vi "probe_calibration.vi"(6 "z offset":sgl=2500.0, 8 "Calibration task":T1, 10 "World light positions":T2 format="%#.1f", 11 "Output pose":dbl[][](array[numeric])) -> (2 "Probe calibration":T2 format="%#.1f")   [LabVIEW 2013]
uses:
  probe_calibration.ctl
  calibration_task.ctl
  <vilib>/Analysis/baseanly.llb/A x Vector.vi
  utilities/labview/norm_vec_single.vi
  <vilib>/Analysis/baseanly.llb/Real A x B.vi
  utilities/labview/norm_vec.vi
  <vilib>/Analysis/baseanly.llb/Real Inverse Matrix.vi
  <vilib>/Analysis/NI_AALBase.lvlib
panel:
  out "Basis":dbl[][](array[numeric])
  # "Construct light calibration from the current light positions.  For the tip lights, this is an initial approximation of the light positions with an arbitrary coordinates based purely on the light locations.  This calibrates for the relative locations of the lights (minimizing triad error.)  With handle lights, the tip coordinates are used to construct the handle coordinates at a fixed Z offset, insuring alignment of the two coordinate systems and eliminating the need for the pivot calibration procedures.  The manipulator must be homed by bottoming it out to force the handle pose into a known relation to the output pose."
  # "This is the offset in microns from light 0  to the origin."
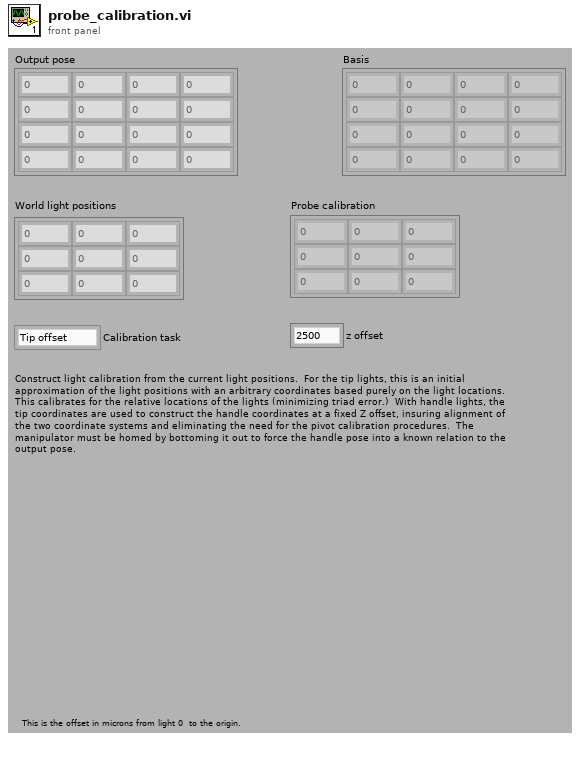
[diagram p1: front panel]
types:
  T1 = typedef "calibration_task.ctl" = enum16{"Tip offset", "RCM offset", "Tip lights", "Handle lights"}
  T2 = typedef "probe_calibration.ctl" = sgl[][]
  T3 = typedef "NI_Matrix.lvlib/RealMatrix.ctl" = dbl[][]
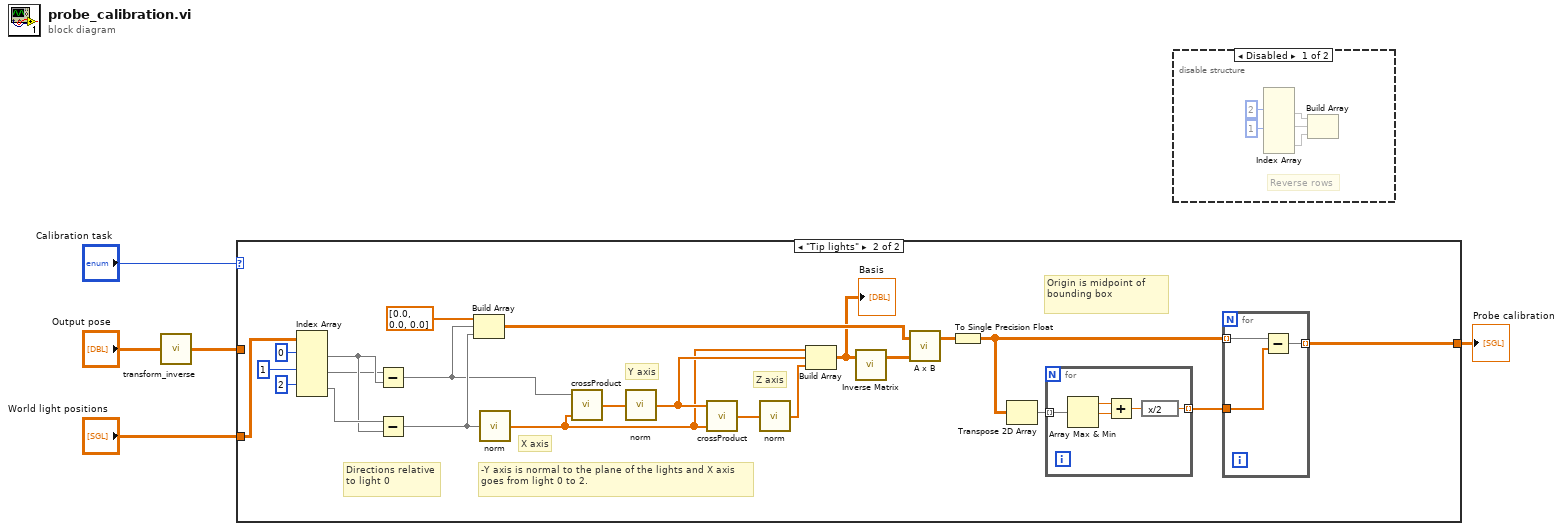
[diagram p0: block diagram]
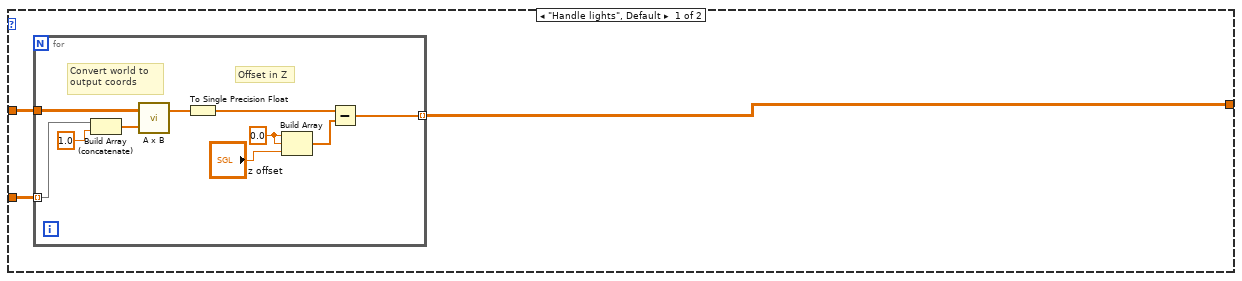
[diagram p3: hidden frame]
diagram:
  n1 = call "transform_inverse.vi"("Transform"="Output pose") -> ("Inverse transform"=w1:T3)
  n2 = case shown="\"Tip lights\"" "Calibration task" {
    tunnel: [w6 w21] -> w5
    tunnel: "World light positions" -> [w8 w27]
    tunnel: w1 -> [w7 _]
    frame "Handle lights", Default {
      n3 = for {
        tunnel: w8 -> [w14] mode=indexing
        tunnel: [w18] -> w6 mode=indexing
        tunnel: w7 -> [w11]
        w16 = sgl 0.0 ("element")
        # "Offset in Z"
        # "Convert world to \noutput coords"
        n4 = Build Array (concatenate)(w14, sgl 1.0) -> (w12:sgl[])
        n5 = call-poly <vilib>:"A x B.vi"("Vector"=w12, "A"=w11) -> ("A x Vector"=w10:dbl[])  [unwired: 1 out]
        n6 = To Single Precision Float(number=w10) -> (single precision float=w9:sgl[])
        n7 = Build Array(w16, w16, "z offset") -> (w15:sgl[])
        n8 = Subtract(x=w9, y=w15) -> (x-y=w18:sgl[])
      }
    }
    frame "Tip lights" {
      # "Origin is midpoint of bounding box"
      # "-Y axis is normal to the plane of the lights and X axis goes from light 0 to 2."
      # "Directions relative to light 0"
      # "Z axis"
      # "Y axis"
      # "X axis"
      n9 = Index Array(array=w27, index (row) #1=0 ("index (row)"), index (row) #2=1 ("index (row)"), index (row) #3=2 ("index (row)")) -> (element #1=w37:sgl[], element #2=w36:sgl[], element #3=w38:sgl[])  [unwired: 3 in]
      n10 = Subtract(x=w36, y=w37) -> (x-y=w20:sgl[])
      n11 = Subtract(x=w38, y=w37) -> (x-y=w31:sgl[])
      n12 = Build Array(dbl[] [0.0, 0.0, 0.0] ("normalized vector"), w20, w31) -> (w30:dbl[][])
      n13 = call-poly "norm.vi"("vector"=w31) -> ("normalized vector"=w19:sgl[])  [unwired: 4 out]
      n14 = call "crossProduct.vi"("B"=w19, "A"=w20) -> ("A x B"=w35:dbl[])  [unwired: 3 out]
      n15 = call-poly "norm.vi"("vector"=w35) -> ("normalized vector"=w23:dbl[])  [unwired: 4 out]
      n16 = call "crossProduct.vi"("B"=w19, "A"=w23) -> ("A x B"=w34:dbl[])  [unwired: 3 out]
      n17 = call-poly "norm.vi"("vector"=w34) -> ("normalized vector"=w33:dbl[])  [unwired: 4 out]
      n18 = Build Array(w19, w23, w33) -> (w22:dbl[][])
      "Basis" <- w22
      n19 = call-poly <vilib>:"Inverse Matrix.vi"("Input Matrix"=w22) -> ("Inverse Matrix"=w28:T3)  [unwired: 1 in, 1 out]
      n20 = call-poly <vilib>:"A x B.vi"("B"=w28, "A"=w30) -> ("A x B"=w29:T3)  [unwired: 1 out]
      n21 = To Single Precision Float(number=w29) -> (single precision float=w25:sgl[][])
      n22 = Transpose 2D Array(2D array=w25) -> (transposed array=w26:sgl[][])
      n23 = for {
        tunnel: w26 -> [w49] mode=indexing
        tunnel: [w45] -> w24 mode=indexing
        n24 = Array Max & Min(array=w49) -> (max value=w48:sgl, min value=w47:sgl)  [unwired: 2 out]
        n25 = Add(x=w48, y=w47) -> (x+y=w46:sgl)
        n26 = expression code="x/2"(w46) -> (w45:sgl)
      }
      n27 = for {
        tunnel: w25 -> [w44] mode=indexing
        tunnel: [w42] -> w21 mode=indexing
        tunnel: w24 -> [w43]
        n28 = Subtract(x=w44, y=w43) -> (x-y=w42:sgl[])
      }
    }
  }
  "Probe calibration" <- w5
  n29 = disable-structure shown="Disabled" {
    frame Disabled {
      # "Reverse rows"
      n30 = Index Array(index (row) #1=2 ("index (row)"), index (row) #2=1 ("index (row)")) -> (array=w50:sgl[][], element #1=w53, element #2=w54, element #3=w55)  [unwired: 4 in]
      n31 = Build Array(w53, w54, w55) -> ()  [unwired: 1 out]
    }
    frame Enabled {
    }
  }
